vi "MultiAxisPositioning.vi"(0 "connection ID":i32, 5 "error in":errorcluster) -> (14 "connection ID":i32, 19 "error out":errorcluster)   [LabVIEW 2016]
doc: "Simultaneously set 3 axes positions\n and get positions to minimize network latency"
panel:
  out "pos3":i32
  out "pos2":i32
  out "pos1":i32
  out "refpos3":i32
  out "refpos2":i32
  out "refpos1":i32
  out "ref3":bool
  out "ref2":bool
  out "ref1":bool
  in  "target3":i32
  in  "target2":i32
  in  "target1":i32
  in  "set3":bool
  in  "set2":bool
  in  "set1":bool
  out "params_cluster":T1
  in  "Params_cluster":T2
  in  "results_cluster":T3
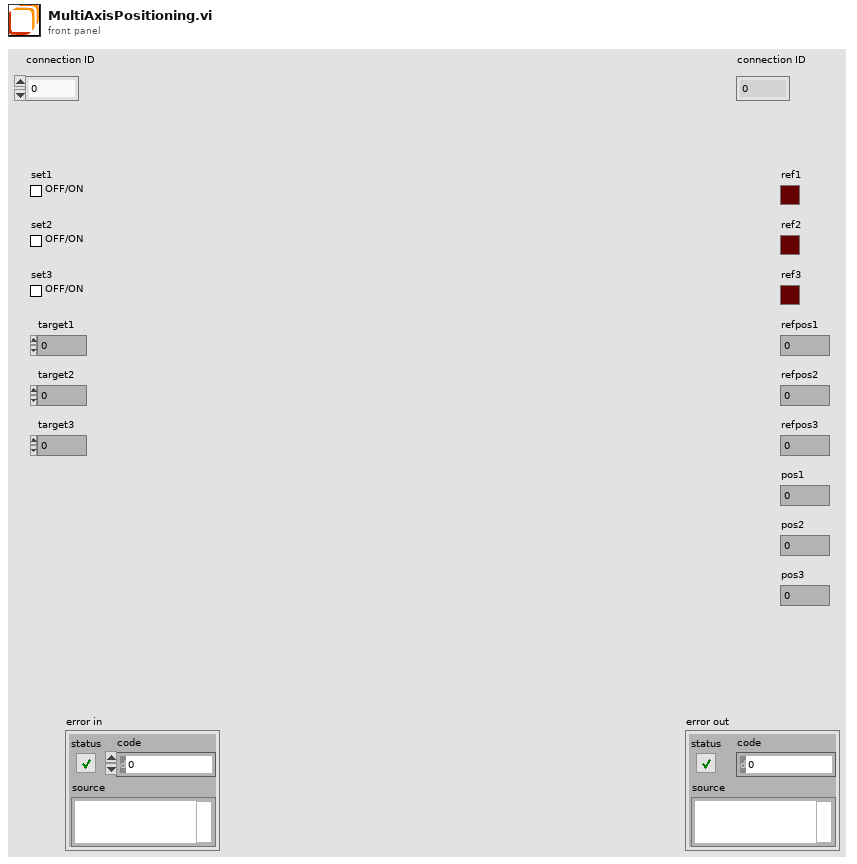
[diagram p1: front panel]
types:
  T1 = cluster{"set1":bool, "set2":bool, "set3":bool, "target1":i32, "target2":i32, "target3":i32}
  T2 = cluster{"boolean":bool, "boolean":bool, "boolean":bool, "integer":i32, "integer":i32, "integer":i32}
  T3 = cluster{"errNo":i32, "ref1":bool, "ref2":bool, "ref3":bool, "refpos1":i32, "refpos2":i32, "refpos3":i32, "pos1":i32, "pos2":i32, "pos3":i32}
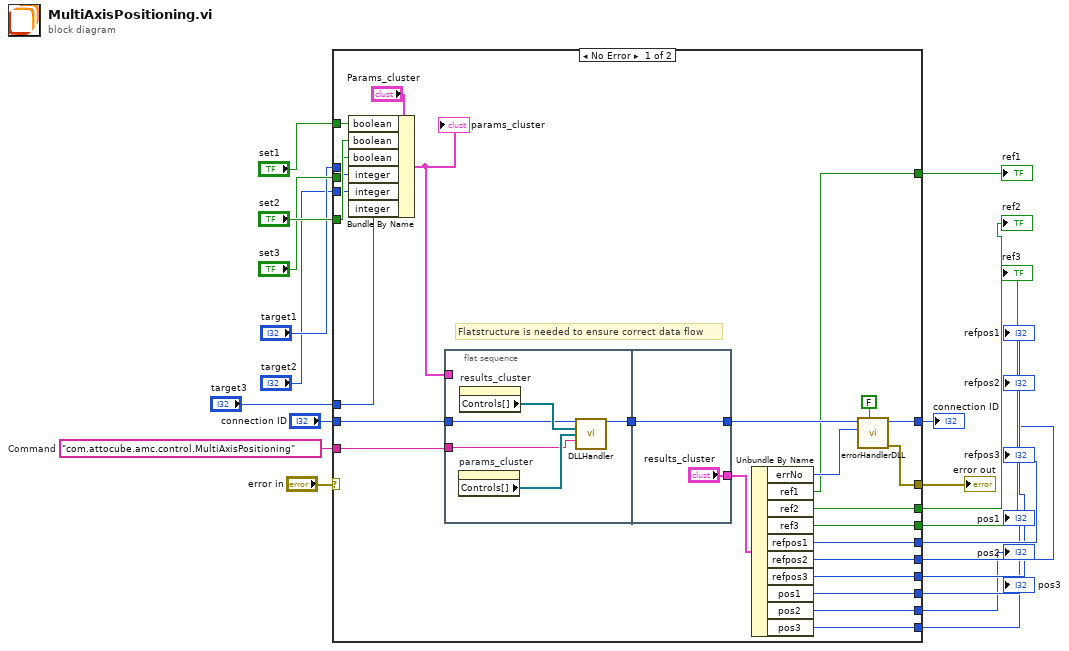
[diagram p0: block diagram]
diagram:
  w18 = "com.attocube.amc.control.MultiAxisPositioning"  # Command
  n1 = case shown="No Error" "error in" {
    selector: "error in" -> [_ w55]
    tunnel: [w45 w55] -> w20
    tunnel: w18 -> [w40 _]
    tunnel: [w39 w54] -> w17
    tunnel: "connection ID" -> [w38 w54]
    tunnel: "set1" -> [w35 _]
    tunnel: "set2" -> [w34 _]
    tunnel: "set3" -> [w33 _]
    tunnel: "target1" -> [w32 _]
    tunnel: "target2" -> [w31 _]
    tunnel: "target3" -> [w30 _]
    tunnel: [w29 _] -> w9
    tunnel: [w28 _] -> w8
    tunnel: [w27 _] -> w7
    tunnel: [w26 _] -> w6
    tunnel: [w25 _] -> w5
    tunnel: [w24 _] -> w4
    tunnel: [w23 _] -> w3
    tunnel: [w22 _] -> w2
    tunnel: [w21 _] -> w1
    frame No Error {
      # "Flatstructure is needed to ensure correct data flow"
      n2 = Bundle By Name(cluster="Params_cluster", "boolean"=w35, "boolean"=w34, "boolean"=w33, "integer"=w32, "integer"=w31, "integer"=w30) -> (w36:T2)
      "params_cluster" <- w36
      n3 = flat-sequence {
        tunnel: [w51] -> w42
        tunnel: w40 -> [w48]
        tunnel: w38 -> [w47]
        tunnel: w36 -> [_]
        tunnel: ["results_cluster"] -> w43
        tunnel: [w53] -> w44
        tunnel: w42 -> [w53]
        frame #0 {
          n4 = property on="params_cluster" class="Clust (strict)"() -> ("Controls[]"=w49:refnum<vi>[])  [unwired: 2 in, 2 out]
          n5 = property on="results_cluster" class="Clust (strict)"() -> ("Controls[]"=w50:refnum<vi>[])  [unwired: 2 in, 2 out]
          n6 = call "DLLHandler.vi"("connection ID"=w47, "results_cluster"=w50, "params_cluster"=w49, "method"=w48) -> ("connection ID out"=w51:i32)  [unwired: 10 in, 1 out]
        }
        frame #1 {
        }
      }
      n7 = Unbundle By Name(w43) -> ("errNo"=w37:i32, "ref1"=w29:bool, "ref2"=w28:bool, "ref3"=w27:bool, "refpos1"=w26:i32, "refpos2"=w25:i32, "refpos3"=w24:i32, "pos1"=w23:i32, "pos2"=w22:i32, "pos3"=w21:i32)
      n8 = call "errorHandlerDLL.vi"("show popup"=FALSE, "error number"=w37, "connection ID"=w44) -> ("error out"=w45:errorcluster, "connection ID"=w39:i32)  [unwired: 7 in]
    }
    frame Error {
    }
  }
  "error out" <- w20
  "connection ID" <- w17
  "ref1" <- w9
  "ref2" <- w8
  "ref3" <- w7
  "refpos1" <- w6
  "refpos2" <- w5
  "refpos3" <- w4
  "pos1" <- w3
  "pos2" <- w2
  "pos3" <- w1
